vi "niDTS WLAN INSTR RX Abort.vi"(8 "error in (no error)":errorcluster, 11 "niDTS WLAN INSTR RX in":refnum<class "niDTS WLAN INSTR RX.lvclass">) -> (0 "error out":errorcluster, 3 "niDTS WLAN INSTR RX out":refnum<class "niDTS WLAN INSTR RX.lvclass">)   [LabVIEW 2015, in "niDTS WLAN.lvlib" / "niDTS WLAN INSTR RX.lvclass"]
uses:
  niDTS WLAN INSTR RX.lvclass
  niDTS WLAN INSTR RX.lvclass/niDTS WLAN INSTR RX.ctl
  RiviInstDriver/niRfsgWlan/Objects/niRfsgWlan.lvclass
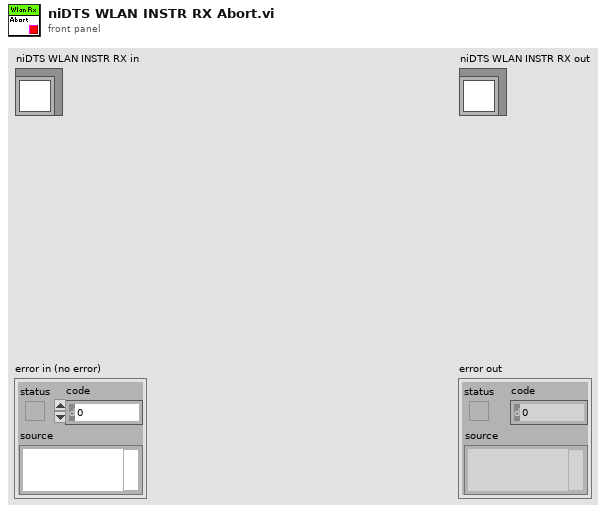
[diagram p1: front panel]
types:
  T1 = typedef "niRfsgWlan.lvclass/niRfsgWlan INC Handle.ctl" = refnum<data-value>
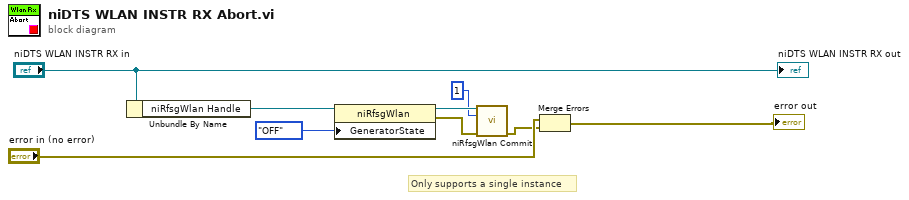
[diagram p0: block diagram]
diagram:
  # "Only supports a single instance"
  n1 = Unbundle By Name("niDTS WLAN INSTR RX in") -> ("niRfsgWlan Handle"=w8:T1)
  n2 = property class="niRfsgWlan"(reference=w8, "GeneratorState"=enum16{"OFF", "PENDING", "ON"}."OFF" ("SOURce:RFSG:WLAN:GeneratorState")) -> (reference out=w6:T1, error out=w5:errorcluster)  [unwired: 1 in]
  n3 = call "niRfsgWlan Commit.vi"("InstDriver Handle in"=w6, "Instance"=1, "error in (no error)"=w5) -> ("error out"=w2:errorcluster)  [unwired: 11 in, 1 out]
  n4 = Merge Errors("error in (no error)", w2) -> (→"error out":errorcluster)
  "niDTS WLAN INSTR RX out" <- "niDTS WLAN INSTR RX in"
